vi "Save to Measurement File_SubVI.vi"(8 "error in (no error)":errorcluster, 11 "Input Cluster Data":T1) -> (0 "error out":errorcluster)   [LabVIEW 2021]
uses:
  Measurement Data Cluster_TDef.ctl
  <vilib>/express/express signal manip/GetorSetDDTAttributes/Shared VIs/TimeType.ctl
  <vilib>/express/express signal manip/GetorSetDDTAttributes/Shared VIs/TimeMode Enum to Boolean.vi
  <vilib>/express/express shared/transition.llb/Dynamic To Waveform Array.vi
  <vilib>/express/express signal manip/GetorSetDDTAttributes/Set DDT Attributes/SetT0.vi
  <vilib>/express/express shared/transition.llb/Waveform Array To Dynamic.vi
  <vilib>/express/express signal manip/GetorSetDDTAttributes/Set DDT Attributes/Set DDT Properties.xnode
  <vilib>/express/express signal manip/GetorSetDDTAttributes/Shared VIs/GetSetShared.lvlib
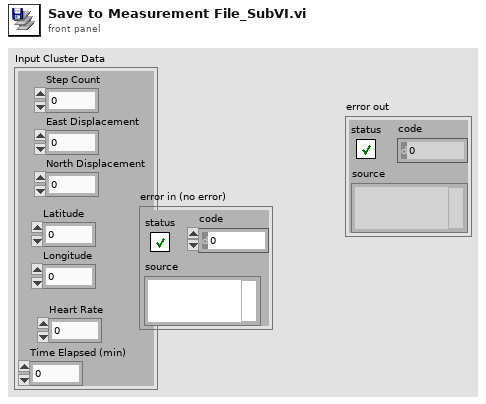
[diagram p1: front panel]
types:
  T1 = typedef "Measurement Data Cluster_TDef.ctl" = cluster{"Step Count":i32, "East Displacement":dbl, "North Displacement":dbl, "Longitude":dbl, "Latitude":dbl, "Heart Rate":dbl, "Time Elapsed (min)":dbl}
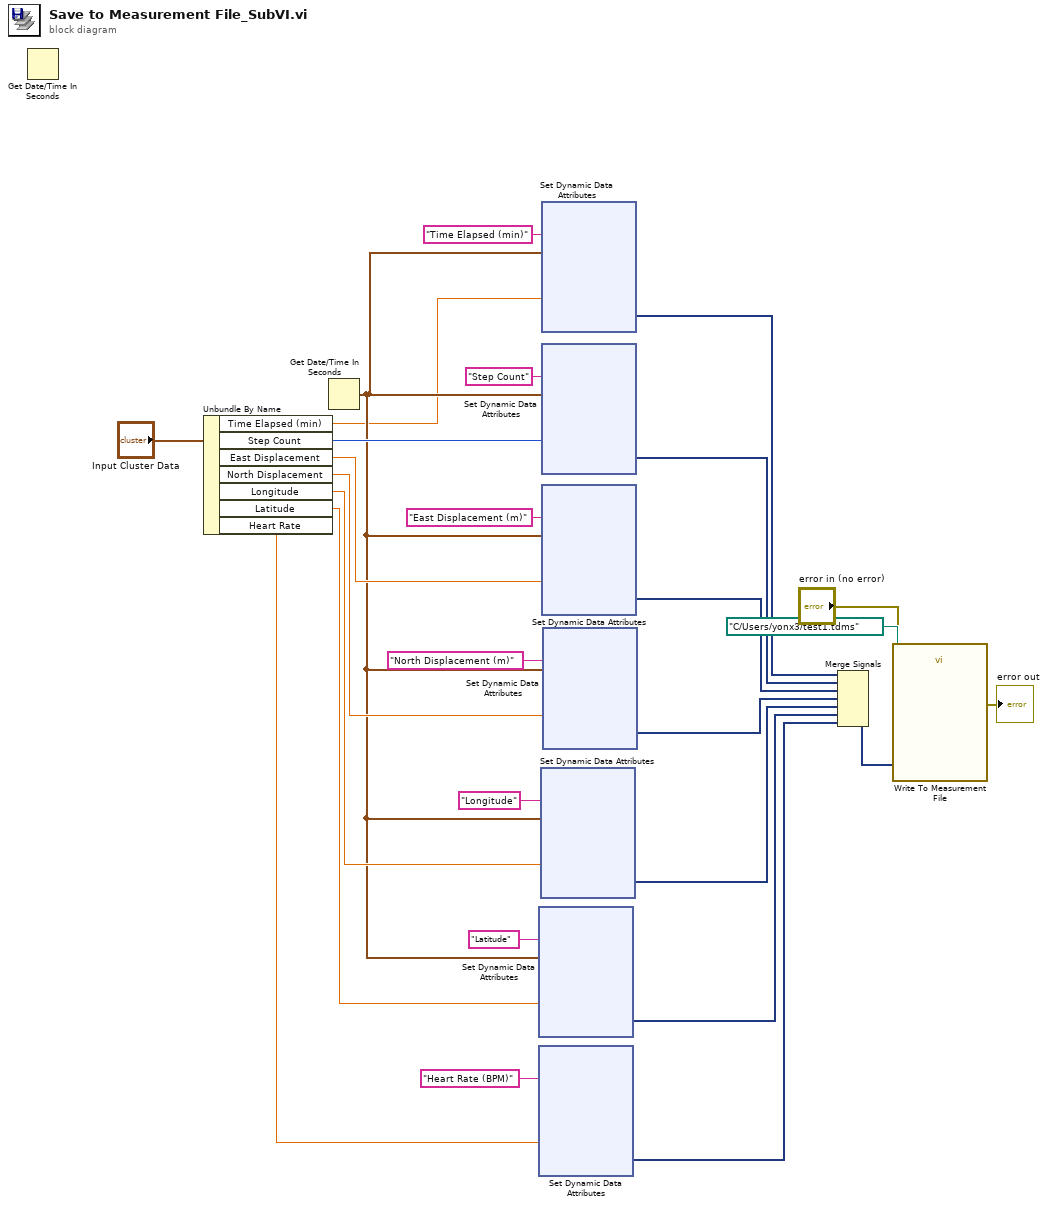
[diagram p0: block diagram]
diagram:
  n1 = Get Date/Time In Seconds() -> ()  [unwired: 1 out]
  n2 = Unbundle By Name("Input Cluster Data") -> ("Time Elapsed (min)"=w4:dbl, "Step Count"=w23:i32, "East Displacement"=w21:dbl, "North Displacement"=w17:dbl, "Longitude"=w16:dbl, "Latitude"=w15:dbl, "Heart Rate"=w2:dbl)
  n3 = Get Date/Time In Seconds() -> (seconds since 1Jan1904=w5:timestamp)
  n4 = xnode "Set Dynamic Data Attributes"("Signals In"=w15, "Signal Name"="Latitude", "Timestamp"=w5) -> ("Signals Out"=w13:dynamicdata)  [unwired: 3 in, 1 out]
  n5 = xnode "Set Dynamic Data Attributes"("Signals In"=w2, "Signal Name"="Heart Rate (BPM)") -> ("Signals Out"=w1:dynamicdata)  [unwired: 4 in, 1 out]
  n6 = xnode "Set Dynamic Data Attributes"("Signals In"=w16, "Signal Name"="Longitude", "Timestamp"=w5) -> ("Signals Out"=w12:dynamicdata)  [unwired: 3 in, 1 out]
  n7 = xnode "Set Dynamic Data Attributes"("Signals In"=w4, "Signal Name"="Time Elapsed (min)", "Timestamp"=w5) -> ("Signals Out"=w6:dynamicdata)  [unwired: 3 in, 1 out]
  n8 = xnode "Set Dynamic Data Attributes"("Signals In"=w23, "Signal Name"="Step Count", "Timestamp"=w5) -> ("Signals Out"=w14:dynamicdata)  [unwired: 3 in, 1 out]
  n9 = xnode "Set Dynamic Data Attributes"("Signals In"=w21, "Signal Name"="East Displacement (m)", "Timestamp"=w5) -> ("Signals Out"=w10:dynamicdata)  [unwired: 3 in, 1 out]
  n10 = xnode "Set Dynamic Data Attributes"("Signals In"=w17, "Signal Name"="North Displacement (m)", "Timestamp"=w5) -> ("Signals Out"=w11:dynamicdata)  [unwired: 2 in, 1 out]
  n11 = Merge Signals(w6, w14, w10, w11, w12, w13, w1) -> (w26:dynamicdata)
  n12 = call "Write To Measurement File"("Signals"=w26, "error in (no error)"="error in (no error)", "Filename"=path "C:/Users/yonx3/test1.tdms") -> ("error out"=→"error out":errorcluster)  [unwired: 14 in, 2 out]
